vi "cRIO_PC_data_transfer.vi"() -> ()   [LabVIEW 2020]
uses:
  <vilib>/WebDAVClient/Advanced/Get File.vi
  <vilib>/WebDAVClient/NI_WebDAV.lvlib
panel:
  out "Transfer Error":errorcluster
  in  "File Name":string
  in  "Save Location (Folder)":path
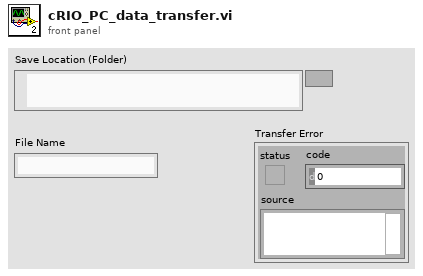
[diagram p1: front panel]
types:
  T1 = typedef "NI_WebDAV.lvlib/SessionHandle.ctl" = refnum<k1>
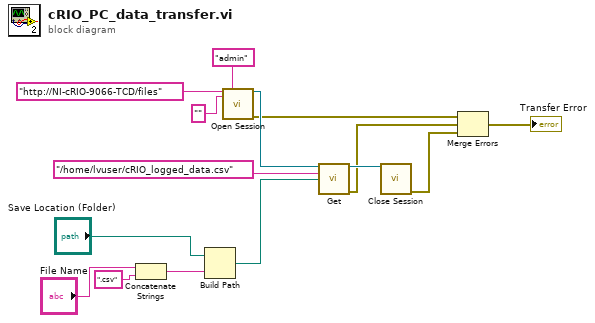
[diagram p0: block diagram]
diagram:
  n1 = Concatenate Strings("File Name", ".csv" ("string")) -> (w6:string)
  n2 = Build Path(base path="Save Location (Folder)", name or relative path=w6) -> (appended path=w5:path)
  n3 = call <vilib>:"Open Session.vi"("host uri prefix"="http://NI-cRIO-9066-TCD/files", "username"="admin", "password"="") -> ("session handle out"=w12:T1, "error out"=w3:errorcluster)  [unwired: 11 in]
  n4 = call-poly <vilib>:"Get.vi"("session handle"=w12, "relative uri"="/home/lvuser/cRIO_logged_data.csv", "local file path"=w5) -> ("session handle out"=w10:T1, "error out"=w2:errorcluster)  [unwired: 10 in, 1 out]
  n5 = call <vilib>:"Close Session.vi"("session handle"=w10) -> ("error out"=w1:errorcluster)  [unwired: 14 in]
  n6 = Merge Errors(w3, w2, w1) -> (→"Transfer Error":errorcluster)
